vi "Test_PublicationLocked_OwnerUnlocks_OK.vi"(8 "error in (no error)":errorcluster, 11 "TestMediator In":refnum<class "TestMediationSemantics.lvclass">) -> (0 "error out":errorcluster, 3 "TestMediator Out":refnum<class "TestMediationSemantics.lvclass">)   [LabVIEW 2020, in "TestMediationSemantics.lvclass"]
uses:
  TestMediationSemantics.lvclass
  TestMediationSemantics.lvclass/TestMediationSemantics.ctl
  Source/Mediator/Mediator/Mediator.lvclass
  <vilib>/ActorFramework/Actor/Actor.lvclass
  Source/IMediator/IMediator Messages/Publish Msg/Publish Msg.lvclass
  Source/IMediator/IMediator Messages/Subscribe Msg/Subscribe Msg.lvclass
  Source/IMediator/SubscriptionRequest/SubscriptionRequest.lvclass
  Source/IMediator/ISubscriptionPolicy/ISubscriptionPolicy.lvclass
  <vilib>/ActorFramework/Stop Msg/Stop Msg.lvclass
  Source/SubscriptionPolicy/BasicSubscription/BasicSubscription.lvclass
  Source/IMediator/IMediator Messages/Lock Publication Msg/Lock Publication Msg.lvclass
  Source/IMediator/IMediator Messages/Unlock Publication Msg/Unlock Publication Msg.lvclass
  modules/composed-transport/Source/Concrete/QueueTransport/QueueTransport.lvclass
  Source/IMediator/PublishRequest/PublishRequest.lvclass
  C:/Git/mva-core/Source/IMediator/IMediator/IMediator.lvclass
  C:/Program Files (x86)/National Instruments/LabVIEW 2020/vi.lib/ActorFramework/Actor/Actor.lvclass
  C:/Git/mva-core/Source/Mediator/Mediator/Mediator.lvclass
  C:/Git/mva-core/Source/IMediator/ISubscriptionPolicy/ISubscriptionPolicy.lvclass
  C:/Git/mva-core/Source/SubscriptionPolicy/BasicSubscription/BasicSubscription.lvclass
  C:/Git/mva-core/modules/composed-transport/Source/ITransport/ITransport.lvclass
  C:/Git/mva-core/modules/composed-transport/Source/Concrete/QueueTransport/QueueTransport.lvclass
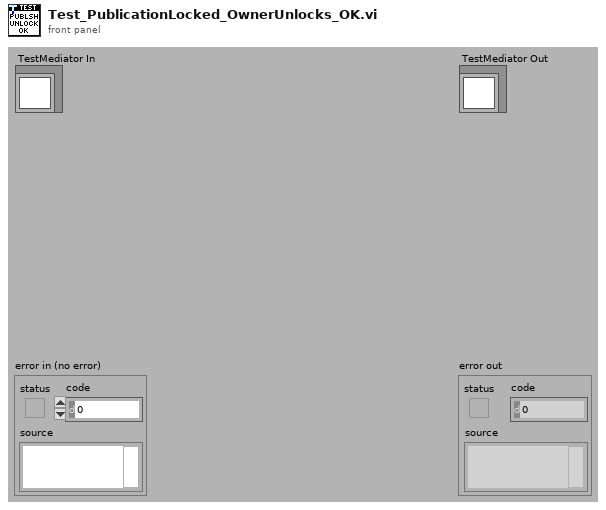
[diagram p1: front panel]
types:
  T1 = typedef "IMediator.lvlib/ISubscriptionPolicy.lvclass/ISubscriptionPolicy Reference.ctl" = refnum<data-value>
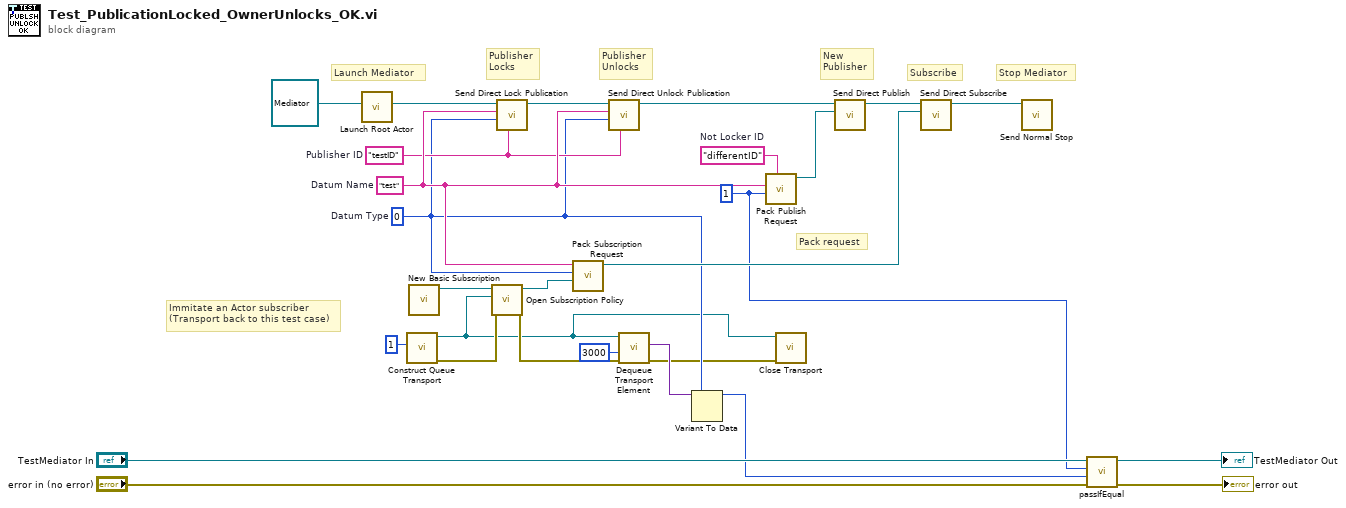
[diagram p0: block diagram]
diagram:
  w10 = "differentID"  # Not Locker ID
  w7 = "testID"  # Publisher ID
  w4 = 0  # Datum Type
  w8 = "test"  # Datum Name
  w3 = 1
  # "Publisher\nUnlocks"
  # "Immitate an Actor subscriber\n(Transport back to this test case)"
  # "Pack request"
  # "Publisher\nLocks"
  # "Launch Mediator"
  # "Stop Mediator"
  # "Subscribe"
  # "New\nPublisher"
  n1 = call <vilib>:"Launch Root Actor.vi"("Actor"=refnum<class "Mediator.lvclass"> refnum ("Mediator.lvlib:Mediator.lvclass")) -> ("Actor's Enqueuer"=w22:refnum<class "Message Enqueuer.lvclass">)  [unwired: 9 in, 1 out]
  n2 = call "Construct Queue Transport.vi"("Max Queue Size (-1)"=1) -> ("error out"=w17:errorcluster, "QueueTransport"=w1:refnum<class "QueueTransport.lvclass">)  [unwired: 9 in]
  n3 = call "New Basic Subscription.vi"() -> ("BasicSubscription Out"=w14:refnum<class "BasicSubscription.lvclass">)  [unwired: 11 in]
  n4 = call "Open Subscription Policy.vi"("error in (no error)"=w17, "Transport"=w1, "SubscriptionPolicy"=w14) -> ("error out"=w16:errorcluster, "Subscription Policy"=w13:T1)  [unwired: 7 in]
  n5 = call "Send Direct Lock Publication.vi"("Publisher ID"=w7, "Datum Type"=w4, "Datum Name"=w8, "Mediator Enqeuer"=w22) -> ("Mediator Enqueuer out"=w11:refnum<class "Message Enqueuer.lvclass">)  [unwired: 6 in, 1 out]
  n6 = call "Pack Subscription Request.vi"("Subscription Policy"=w13, "Type"=w4, "Datum Name"=w8) -> ("SubscriptionRequest"=w21:refnum<class "SubscriptionRequest.lvclass">)  [unwired: 7 in, 1 out]
  n7 = call "Send Direct Unlock Publication.vi"("Publisher ID"=w7, "Datum Type"=w4, "Datum Name"=w8, "Mediator Enqeuer"=w11) -> ("Mediator Enqueuer out"=w9:refnum<class "Message Enqueuer.lvclass">)  [unwired: 6 in, 1 out]
  n8 = call "Dequeue Transport Element.vi"("error in (no error)"=w16, "Timeout In ms (-1)"=3000, "QueueTransport"=w1) -> ("error out"=w2:errorcluster, "Data"=w6:variant)  [unwired: 5 in, 2 out]
  n9 = Variant To Data(type=w4, Variant=w6) -> (data=w5:i32)  [unwired: 1 in, 1 out]
  n10 = call "Pack Publish Request.vi"("Publisher ID"=w10, "Value"=w3, "Datum Name"=w8) -> ("PublishRequest Out"=w12:refnum<class "PublishRequest.lvclass">)  [unwired: 7 in, 1 out]
  n11 = call-dynamic "Close Transport.vi"("error in (no error)"=w2, "QueueTransport"=w1) -> ()  [unwired: 9 in, 1 out]
  n12 = call "Send Direct Publish.vi"("PublishRequest"=w12, "Mediator Enqueuer"=w9) -> ("Mediator Enqueuer out"=w20:refnum<class "Message Enqueuer.lvclass">)  [unwired: 8 in, 1 out]
  n13 = call "Send Direct Subscribe.vi"("Subscription Request"=w21, "Message Enqueuer"=w20) -> ("Message Enqueuer out"=w15:refnum<class "Message Enqueuer.lvclass">)  [unwired: 8 in, 1 out]
  n14 = call <vilib>:"Send Normal Stop.vi"("Message Enqueuer"=w15) -> ()  [unwired: 10 in, 1 out]
  n15 = call-dynamic "passIfEqual.vi"("error in (no error)"="error in (no error)", "y"=w5, "x"=w3, "TestCase in"="TestMediator In") -> ("error out"=→"error out":errorcluster, "TestCase out"=→"TestMediator Out":refnum<class "TestMediationSemantics.lvclass">)  [unwired: 6 in]
